vi "LAC pharse ErrMsg (SubVI).vi"(8 "error in":errorcluster, 10 "Response":string[](array[string]), 11 "VISA resource name":refnum<visa-resource-name>) -> (0 "error out":errorcluster, 2 "ERR?":bool, 3 "VISA resource name out":refnum<visa-resource-name>)   [LabVIEW 2018]
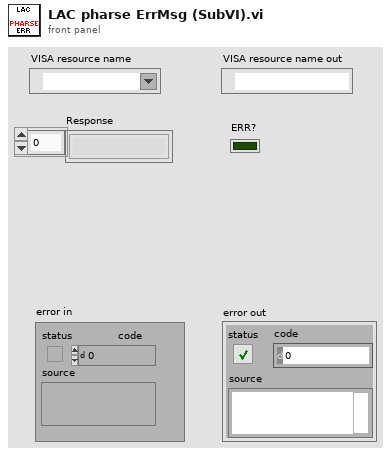
[diagram p1: front panel]
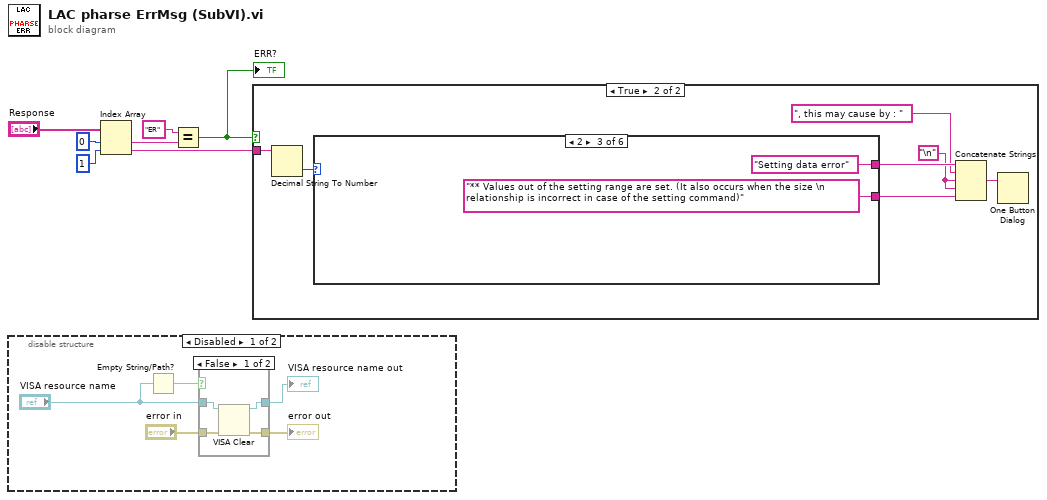
[diagram p0: block diagram]
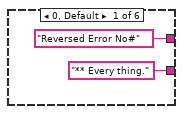
[diagram p3: hidden frame]
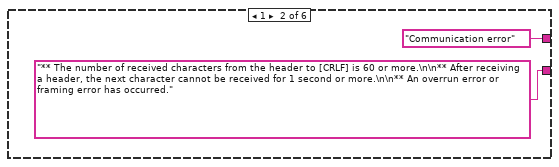
[diagram p4: hidden frame]
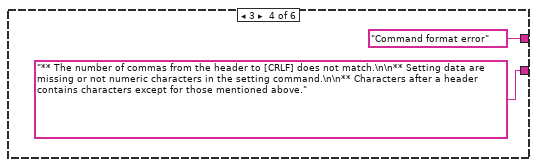
[diagram p5: hidden frame]
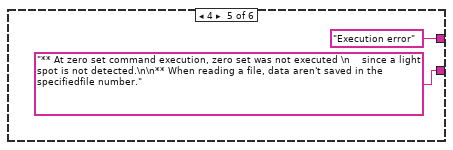
[diagram p6: hidden frame]
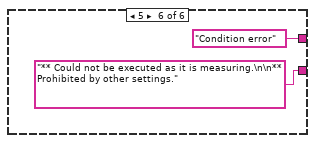
[diagram p7: hidden frame]
diagram:
  n1 = disable-structure shown="Disabled" {
    frame Disabled {
      n2 = Empty String/Path?(string/path="VISA resource name") -> (empty?=w8:bool)
      n3 = case shown="False" w8 {
        tunnel: "error in" -> [w16 w17]
        tunnel: [w15 w18] -> w11
        tunnel: [w14 w17] -> w10
        tunnel: "VISA resource name" -> [w13 w18]
        frame False {
          n4 = VISA Clear(VISA resource name=w13, error in (no error)=w16) -> (VISA resource name out=w15:refnum<visa-resource-name>, error out=w14:errorcluster)
        }
        frame True {
        }
      }
      "VISA resource name out" <- w11
      "error out" <- w10
    }
    frame Enabled {
    }
  }
  n5 = Index Array(array="Response", index #1=0 ("index"), index #2=1 ("index")) -> (element #1=w4:string, element #2=w5:string)
  n6 = Equal?(x="ER", y=w4) -> (x = y?=w1:bool)
  "ERR?" <- w1
  n7 = case shown="True" w1 {
    tunnel: w5 -> [_ w19]
    frame False {
    }
    frame True {
      w20 = "\n"
      n8 = Decimal String To Number(string=w19) -> (number=w21:i32)  [unwired: 2 in, 1 out]
      n9 = case shown="2" w21 {
        tunnel: ["Reversed Error No#" "Communication error" "Setting data error" "Command format error" "Execution error" "Condition error"] -> w23
        tunnel: ["** Every thing." "** The number of received characters from the header to [CRLF] is 60 or more.\n\n** After receiving a header, the next character cannot be received for 1 second or more.\n\n** An overrun error or framing error has occurred." "** Values out of the setting range are set. (It also occurs when the size \n    relationship is incorrect in case of the setting command)" "** The number of commas from the header to [CRLF] does not match.\n\n** Setting data are missing or not numeric characters in the setting command.\n\n** Characters after a header contains characters except for those mentioned above." "** At zero set command execution, zero set was not executed \n    since a light spot is not detected.\n\n** When reading a file, data aren't saved in the specifiedfile number." "** Could not be executed as it is measuring.\n\n** Prohibited by other settings."] -> w24
        frame 0, Default {
        }
        frame 1 {
        }
        frame 2 {
        }
        frame 3 {
        }
        frame 4 {
        }
        frame 5 {
        }
      }
      n10 = Concatenate Strings(w23, ", this may cause by : " ("string"), w20, w20, w24) -> (w25:string)
      n11 = One Button Dialog(message=w25) -> ()  [unwired: 1 in, 1 out]
    }
  }
